vi "Verify Parameters.vi"(8 "error in (no error)":errorcluster, 10 "Parameters In":variant, 11 "SqlMapper in":refnum<class "SqlMapper.lvclass">) -> (0 "error out":errorcluster, 2 "DynamicParameters out":refnum<class "DynamicParameters.lvclass">, 3 "SqlMapper out":refnum<class "SqlMapper.lvclass">)   [LabVIEW 2020, in "ORM_API.lvlib"]
uses:
  ORM_API.lvlib
  <vilib>/Viviota/shared/ORM.lvlibp/ORM/DynamicParameters/DynamicParameters.lvclass
  <vilib>/Viviota/shared/ORM.lvlibp/ORM/SqlMapper/SqlMapper.lvclass
  <vilib>/Viviota/shared/ORM.lvlibp/ORM/TypeMap/TypeMap.lvclass
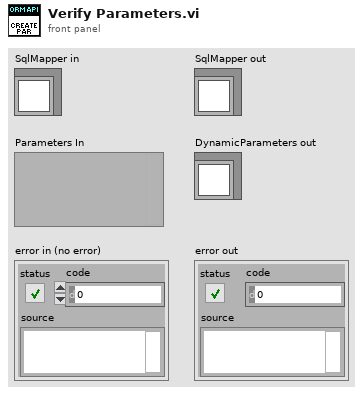
[diagram p1: front panel]
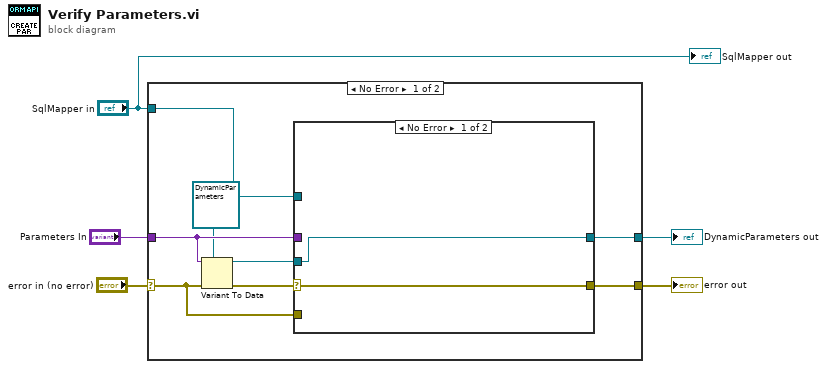
[diagram p0: block diagram]
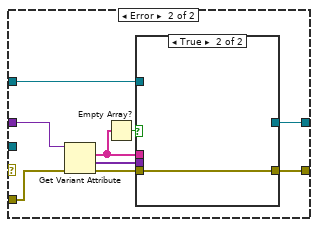
[diagram p2: hidden frame]
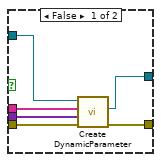
[diagram p3: hidden frame]
diagram:
  n1 = case shown="No Error" "error in (no error)" {
    selector: "error in (no error)" -> [w7 w32]
    tunnel: [w13 w32] -> w5
    tunnel: [w12 _] -> w4
    tunnel: "SqlMapper in" -> [w11 _]
    tunnel: "Parameters In" -> [w9 _]
    frame No Error {
      n2 = Variant To Data(error in=w7, type=refnum<class "DynamicParameters.lvclass"> refnum ("Parameters"), Variant=w9) -> (data=w6:refnum<class "DynamicParameters.lvclass">, error out=w10:errorcluster)
      n3 = case shown="No Error" w10 {
        selector: w10 -> [w14 _]
        tunnel: [w14 w24] -> w13
        tunnel: [w15 w23] -> w12
        tunnel: w9 -> [_ w22]
        tunnel: w11 -> [_ w21]
        tunnel: w7 -> [_ w18]
        tunnel: w6 -> [w15 _]
        frame No Error {
        }
        frame Error {
          n4 = Get Variant Attribute(Variant=w22, error in=w18) -> (names=w17:string[], values=w19:variant[], error out=w20:errorcluster)  [unwired: 2 in, 1 out]
          n5 = Empty Array?(array=w17) -> (empty?=w16:bool)
          n6 = case shown="True" w16 {
            tunnel: [w30 w31] -> w24
            tunnel: [w29 _] -> w23
            tunnel: w21 -> [w28 _]
            tunnel: w20 -> [w27 w31]
            tunnel: w19 -> [w26 _]
            tunnel: w17 -> [w25 _]
            frame False {
              n7 = call <vilib>:"Create DynamicParameter.vi"("error in (no error)"=w27, "ParameterValues"=w26, "ParameterNames"=w25, "SqlMapper in"=w28) -> ("error out"=w30:errorcluster, "Parameters"=w29:refnum<class "DynamicParameters.lvclass">)  [unwired: 3 in, 3 out]
            }
            frame True {
            }
          }
        }
      }
    }
    frame Error {
    }
  }
  "error out" <- w5
  "DynamicParameters out" <- w4
  "SqlMapper out" <- "SqlMapper in"
